vi "Begin.vi"(8 "error in":errorcluster) -> (0 "error out":errorcluster)   [LabVIEW 2018]
doc: "Called before other user functions, this VI is expected to open initial I/O refnums, load in file data, and do all program initialization. Notice that the <B>error out</B> terminal is simply used for data flow. Wiring it to other structures or subVIs ensures that this VI runs first."
uses:
  <vilib>/Rock Robotics/WPI/DriverStation/WPI_DriverStationRobotMode2.ctl
  <vilib>/Rock Robotics/SystemInterfaces/DIO/FPGA_DIOChannel.ctl
  <vilib>/Rock Robotics/SystemInterfaces/DIO/FPGA_DIOPWMChannel.ctl
  <vilib>/Rock Robotics/WPI/Joystick/WPI_JoystickDeviceEnum.ctl
  <vilib>/Rock Robotics/WPI/SafetyOutput/WPI_SafetyOutputConfigMenu.ctl
  <vilib>/Rock Robotics/WPI/Solenoid/WPI_SolenoidChannel.ctl
  <vilib>/Rock Robotics/WPI/Solenoid/WPI_SolenoidValue.ctl
  <vilib>/Rock Robotics/WPI/ThirdParty/Phoenix-LabVIEW/Motor Controller/Controls/CTRE_Phoenix_MotorControl_FeedbackDevice.ctl
  Robot Global Data.vi
  <vilib>/Rock Robotics/Network Tables/NT Write String Array.vi
  <vilib>/Rock Robotics/Network Tables/NT Write Number.vi
  Refnums.vi
  CAN ID's.vi
  <vilib>/Rock Robotics/WPI/RobotDrive/WPI_RobotDriveOpen2MotorWithExistingMotors.vi
  <vilib>/Rock Robotics/WPI/Solenoid/WPI_SolenoidOpenDouble.vi
  <vilib>/Rock Robotics/WPI/Solenoid/WPI_SolenoidSetEnum.vi
  <vilib>/Rock Robotics/WPI/Utilities/WPI_GetSetVariantRefNum.vi
  PID Values.vi
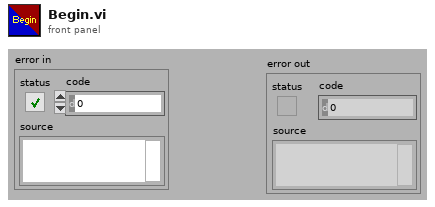
[diagram p1: front panel]
types:
  T1 = typedef "WPI_DriverStationRobotMode2.ctl" = enum16{"Autonomous Disabled", "Autonomous Enabled", "Teleop Disabled", "Teleop Enabled", "Disconnected", "Finish", "Test Disabled", "Test Enabled", "Emergency Stopped"}
  T2 = typedef "WPI_JoystickDeviceEnum.ctl" = enum16{"USB 0", "USB 1", "USB 2", "USB 3", "USB 4", "USB 5"}
  T3 = typedef "FPGA_DIOPWMChannel.ctl" = enum8{"PWM 0", "PWM 1", "PWM 2", "PWM 3", "PWM 4", "PWM 5", "PWM 6", "PWM 7", "PWM 8", "PWM 9", "PWM MXP 0", "PWM MXP 1", "PWM MXP 2", "PWM MXP 3", "PWM MXP 4", "PWM MXP 5", "PWM MXP 6", "PWM MXP 7", "PWM MXP 8", "PWM MXP 9", "Invalid"}
  T4 = typedef "FPGA_DIOChannel.ctl" = enum8{"DIO 0", "DIO 1", "DIO 2", "DIO 3", "DIO 4", "DIO 5", "DIO 6", "DIO 7", "DIO 8", "DIO 9", "DIO MXP 0", "DIO MXP 1", "DIO MXP 2", "DIO MXP 3", "DIO MXP 4", "DIO MXP 5", "DIO MXP 6", "DIO MXP 7", "DIO MXP 8", "DIO MXP 9", "DIO MXP 10", "DIO MXP 11", "DIO MXP 12", "DIO MXP 13", "DIO MXP 14", "DIO MXP 15", "SPI Port CS1", "SPI Port CS2", "SPI Port CS3", "SPI Port MISO", "SPI Port MOSI", "Invalid"}
  T5 = typedef "WPI_SafetyOutputConfigMenu.ctl" = enum16{"Enable", "Disable"}
  T6 = typedef "WPI_SolenoidValue.ctl" = enum16{"Off", "On", "Forward", "Reverse"}
  T7 = typedef "WPI_SolenoidChannel.ctl" = enum8{"Solenoid 0", "Solenoid 1", "Solenoid 2", "Solenoid 3", "Solenoid 4", "Solenoid 5", "Solenoid 6", "Solenoid 7", "Invalid"}
  T8 = typedef "WPI_ServoDeviceRef.ctl" = cluster{"DeviceStatus":errorcluster, "PWM Channel":T3, "DeadBand":T9}
  T9 = typedef "WPI_PWMDeadband.ctl" = cluster{"Name":string, "maxPositivePwm":i32, "minPositivePwm":i32, "centerPwm":i32, "maxNegativePwm":i32, "minNegativePwm":i32, "angularRange":u16}
  T10 = typedef "WPI_JoystickDevRef.ctl" = cluster{"Device":T2}
  T11 = typedef "WPI_DigitalInputDevRef.ctl" = cluster{"DevStatus":errorcluster, "DIO Channel":T4}
  T12 = typedef "WPI_MotorControlDeviceRef.ctl" = cluster{"DeviceStatus":errorcluster, "Type":T13, "PWM":cluster{"PWM Channel":T3, "DeadBand":T9}, "CAN":cluster{"Device Number":u8, "SetOutput VI Ref":variant, "GetOutput VI Ref":variant, "Enable VI Ref":variant, "Disable VI Ref":variant, "Data":variant}, "Invert":bool, "DIO PWM":cluster{"PWM \"Enable\" Channel":T3, "DIOChannel":T4, "PWM Rate":dbl}}
  T13 = typedef "WPI_MotorControlType.ctl" = enum16{"PWM", "CAN", "DIO PWM"}
  T14 = typedef "WPI_RobotDriveDevRef.ctl" = cluster{"DevStatus":errorcluster, "Motors[]":T12[], "Square Inputs":bool, "Max Output":dbl}
  T15 = typedef "WPI_SolenoidDevRef.ctl" = cluster{"DevStatus":errorcluster, "Pneumatics Control Module":u8, "Forward Solenoid Channel":T7, "Reverse Solenoid Channel":T7}
  T16 = typedef "WPI_CompressorDevRef.ctl" = cluster{"DevStatus":errorcluster, "Pneumatics Control Module":u8}
  T17 = cluster{"DriveShifter":T15, "Ouput":T15, "Compressor":T16, "Climb Piston":T15}
  T18 = typedef "CTRE_Phoenix_MotorControl_FeedbackDevice.ctl" = i8
  T19 = cluster{"P":dbl, "I":dbl, "D":dbl, "F":dbl, "I Zone":dbl}
  T20 = cluster{"RightMaster":u8, "RightSlaveA":u8, "RightSlaveB":u8, "LeftMaster":u8, "LeftSlaveA":u8, "LeftSlaveB":u8, "PCM":u8, "PDP":u8, "Intake":u8, "Pivot":u8, "Elevator":u8, "Right Climber":u8, "Left Climber":u8, "Shooter":u8}
  T21 = cluster{"DriveTrain":T14, "LeftDrive":T12, "RightDrive":T12, "Elevator":T12, "Pivot":T12, "Intake":T12, "Right Climber":T12, "Left Climber":T12, "Shooter":T12}
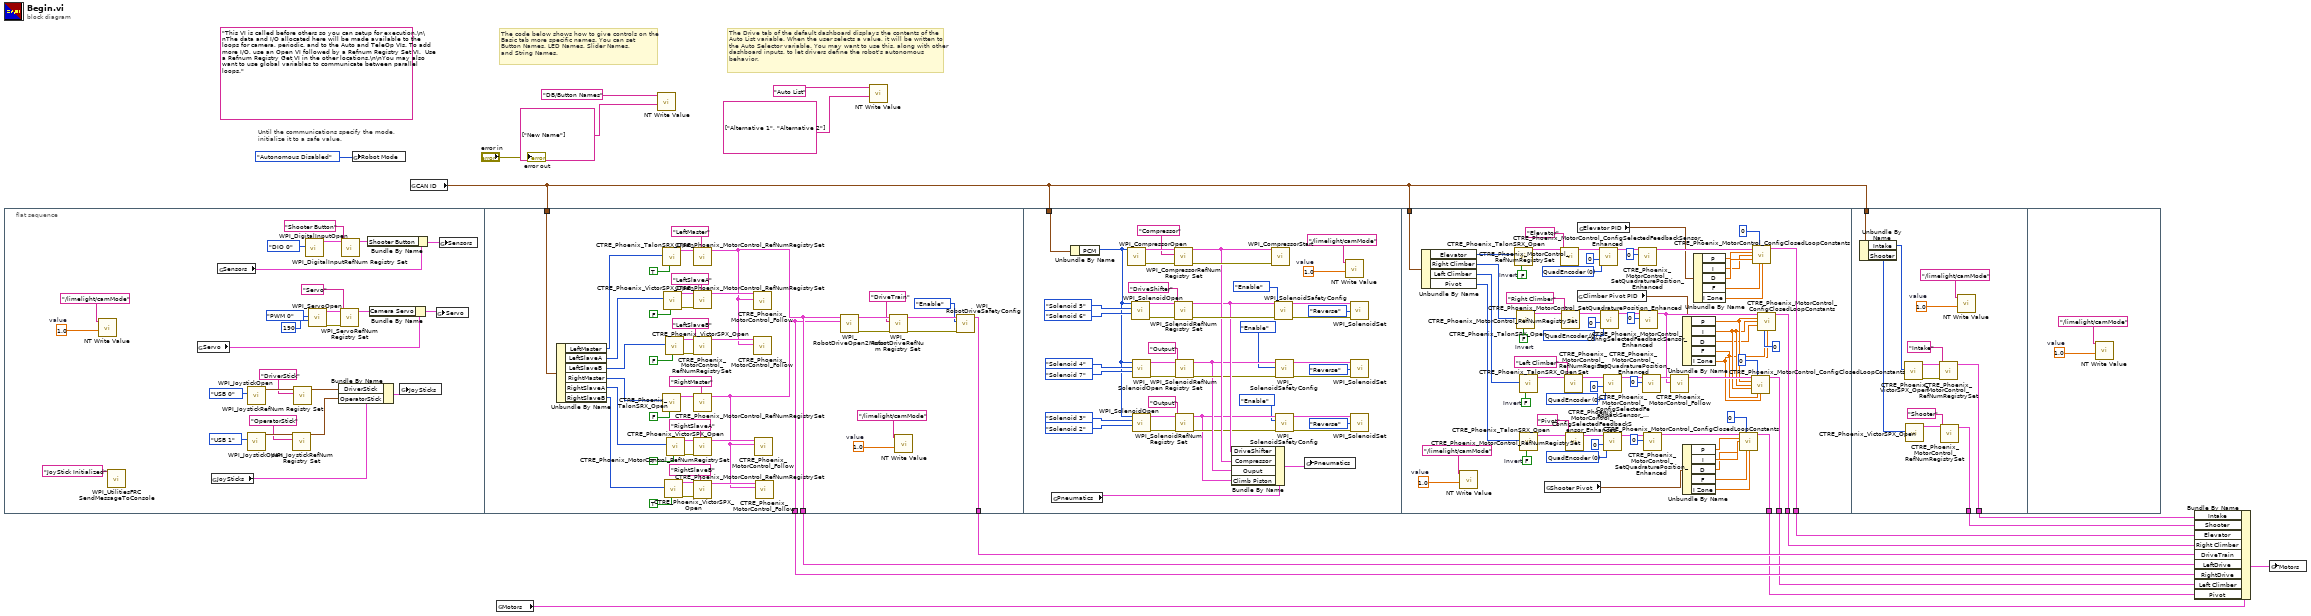
[diagram p0: block diagram]
diagram:
  (unwired) "This VI is called before others so you can setup for execution.\n\nThe data and I/O allocated here will be made available to the loops for camera, periodic, and to the Auto and TeleOp VIs. To add more I/O, use an Open VI followed by a Refnum Registry Set VI.  Use a Refnum Registry Get VI in the other locations.\n\nYou may also want to use global variables to communicate between parallel loops."
  # "The Drive tab of the default dashboard displays the contents of the\nAuto List variable. When the user selects a value, it will be written to\nthe Auto Selector variable. You may want to use this, along with other\ndashboard inputs, to let drivers define the robot's autonomous\nbehavior."
  # "The code below shows how to give controls on the\nBasic tab more specific names. You can set\nButton Names, LED Names, Slider Names,\nand String Names."
  # "Until the communications specify the mode,\ninitialize it to a safe value."
  n1 = flat-sequence {
    tunnel: w3 -> [w69]
    tunnel: [w68] -> w11
    tunnel: [w67] -> w10
    tunnel: [w66] -> w9
    tunnel: w3 -> [w118]
    tunnel: w3 -> [w203]
    tunnel: [w159] -> w7
    tunnel: [w150] -> w6
    tunnel: [w164] -> w5
    tunnel: [w163] -> w4
    tunnel: w3 -> [w210]
    tunnel: [w207] -> w2
    tunnel: [w206] -> w1
    frame #0 {
      w19 = 1.0  # value
      n2 = call-poly <vilib>:"NT Write Value.vi"("Numeric"=w19, "Name"="/limelight/camMode") -> ()  [unwired: 9 in, 1 out]
      n3 = call <vilib>:"WPI_UtilitiesFRC SendMessageToConsole.vi"("Message"="JoyStick Initialized") -> ()  [unwired: 14 in, 1 out]
      n4 = global read "Refnums.vi" "Servo"() -> (w28:cluster{"Camera Servo":T8})
      n5 = global read "Refnums.vi" "JoySticks"() -> (w43:cluster{"DriverStick":T10, "OperatorStick":T10})
      n6 = global read "Refnums.vi" "Sensors"() -> (w31:cluster{"Shooter Button":T11})
      n7 = call <vilib>:"WPI_JoystickOpen.vi"("JoystickDevice"=WPI_JoystickDeviceEnum."USB 1") -> ("JoystickDevRef"=w25:T10)  [unwired: 10 in]
      n8 = call <vilib>:"WPI_JoystickOpen.vi"("JoystickDevice"=WPI_JoystickDeviceEnum."USB 0") -> ("JoystickDevRef"=w45:T10)  [unwired: 10 in]
      n9 = call <vilib>:"WPI_JoystickRefNum Registry Set.vi"("refnum name"="OperatorStick", "JoystickDevRef"=w25) -> ("JoystickDevRef"=w23:T10)  [unwired: 8 in, 1 out]
      n10 = call <vilib>:"WPI_JoystickRefNum Registry Set.vi"("refnum name"="DriverStick", "JoystickDevRef"=w45) -> ("JoystickDevRef"=w42:T10)  [unwired: 8 in, 1 out]
      n11 = call <vilib>:"WPI_DigitalInputOpen.vi"("DIO Channel"=FPGA_DIOChannel."DIO 0") -> ("DigitalInputDevRef"=w38:T11)  [unwired: 9 in, 1 out]
      n12 = call <vilib>:"WPI_ServoOpen.vi"("Angular Range"=u16 190, "PWM Channel"=FPGA_DIOPWMChannel."PWM 0") -> ("error out"=w34:errorcluster, "ServoDeviceRef"=w33:T8)  [unwired: 8 in]
      n13 = Bundle By Name(cluster=w43, "DriverStick"=w42, "OperatorStick"=w23) -> (w41:cluster{"DriverStick":T10, "OperatorStick":T10})
      n14 = call <vilib>:"WPI_ServoRefNum Registry Set.vi"("error in (no error)"=w34, "refnum name"="Servo", "ServoDeviceRef"=w33) -> ("ServoDeviceRef"=w27:T8)  [unwired: 7 in, 1 out]
      n15 = call <vilib>:"WPI_DigitalInputRefNum Registry Set.vi"("refnum name"="Shooter Button", "DigitalInputDevRef"=w38) -> ("DigitalInputDevRef"=w30:T11)  [unwired: 8 in, 1 out]
      n16 = Bundle By Name(cluster=w31, "Shooter Button"=w30) -> (w29:cluster{"Shooter Button":T11})
      n17 = Bundle By Name(cluster=w28, "Camera Servo"=w27) -> (w26:cluster{"Camera Servo":T8})
      n18 = global write "Refnums.vi" "JoySticks"(w41) -> ()
      n19 = global write "Refnums.vi" "Servo"(w26) -> ()
      n20 = global write "Refnums.vi" "Sensors"(w29) -> ()
    }
    frame #1 {
      w46 = 1.0  # value
      n21 = Unbundle By Name(w69) -> ("LeftMaster"=w82:u8, "LeftSlaveA"=w53:u8, "LeftSlaveB"=w52:u8, "RightMaster"=w80:u8, "RightSlaveA"=w51:u8, "RightSlaveB"=w50:u8)
      n22 = call <vilib>:"CTRE_Phoenix_TalonSRX_Open.vi"("Invert"=TRUE, "Device Number"=w82) -> ("CAN Talon SRX Ref"=w83:T12)  [unwired: 8 in, 1 out]
      n23 = call <vilib>:"CTRE_Phoenix_TalonSRX_Open.vi"("Invert"=FALSE, "Device Number"=w80) -> ("CAN Talon SRX Ref"=w81:T12)  [unwired: 8 in, 1 out]
      n24 = call <vilib>:"CTRE_Phoenix_VictorSPX_Open.vi"("Invert"=FALSE, "Device Number"=w53) -> ("error out"=w63:errorcluster, "CAN Talon SRX Ref"=w62:T12)  [unwired: 8 in]
      n25 = call <vilib>:"CTRE_Phoenix_VictorSPX_Open.vi"("Invert"=TRUE, "Device Number"=w50) -> ("error out"=w57:errorcluster, "CAN Talon SRX Ref"=w56:T12)  [unwired: 8 in]
      n26 = call <vilib>:"CTRE_Phoenix_VictorSPX_Open.vi"("Invert"=FALSE, "Device Number"=w52) -> ("error out"=w61:errorcluster, "CAN Talon SRX Ref"=w60:T12)  [unwired: 8 in]
      n27 = call <vilib>:"CTRE_Phoenix_VictorSPX_Open.vi"("Invert"=TRUE, "Device Number"=w51) -> ("error out"=w59:errorcluster, "CAN Talon SRX Ref"=w58:T12)  [unwired: 8 in]
      n28 = call <vilib>:"CTRE_Phoenix_MotorControl_RefNumRegistrySet.vi"("refnum name"="LeftMaster", "PhoenixMotorControlDevRef"=w83) -> ("PhoenixMotorControlDevRef"=w67:T12)  [unwired: 8 in, 1 out]
      n29 = call <vilib>:"CTRE_Phoenix_MotorControl_RefNumRegistrySet.vi"("error in (no error)"=w63, "refnum name"="LeftSlaveA", "PhoenixMotorControlDevRef"=w62) -> ("PhoenixMotorControlDevRef"=w78:T12)  [unwired: 7 in, 1 out]
      n30 = call <vilib>:"CTRE_Phoenix_MotorControl_RefNumRegistrySet.vi"("error in (no error)"=w61, "refnum name"="LeftSlaveB", "PhoenixMotorControlDevRef"=w60) -> ("PhoenixMotorControlDevRef"=w79:T12)  [unwired: 7 in, 1 out]
      n31 = call <vilib>:"CTRE_Phoenix_MotorControl_RefNumRegistrySet.vi"("refnum name"="RightMaster", "PhoenixMotorControlDevRef"=w81) -> ("PhoenixMotorControlDevRef"=w66:T12)  [unwired: 8 in, 1 out]
      n32 = call <vilib>:"CTRE_Phoenix_MotorControl_RefNumRegistrySet.vi"("error in (no error)"=w59, "refnum name"="RightSlaveA", "PhoenixMotorControlDevRef"=w58) -> ("PhoenixMotorControlDevRef"=w77:T12)  [unwired: 7 in, 1 out]
      n33 = call <vilib>:"CTRE_Phoenix_MotorControl_RefNumRegistrySet.vi"("error in (no error)"=w57, "refnum name"="RightSlaveB", "PhoenixMotorControlDevRef"=w56) -> ("PhoenixMotorControlDevRef"=w76:T12)  [unwired: 7 in, 1 out]
      n34 = call <vilib>:"CTRE_Phoenix_MotorControl_Follow.vi"("Master Controller to Follow"=w67, "PhoenixMotorControlDevRef"=w78) -> ()  [unwired: 8 in, 2 out]
      n35 = call <vilib>:"CTRE_Phoenix_MotorControl_Follow.vi"("Master Controller to Follow"=w67, "PhoenixMotorControlDevRef"=w79) -> ()  [unwired: 8 in, 2 out]
      n36 = call <vilib>:"CTRE_Phoenix_MotorControl_Follow.vi"("Master Controller to Follow"=w66, "PhoenixMotorControlDevRef"=w77) -> ()  [unwired: 8 in, 2 out]
      n37 = call <vilib>:"CTRE_Phoenix_MotorControl_Follow.vi"("Master Controller to Follow"=w66, "PhoenixMotorControlDevRef"=w76) -> ()  [unwired: 8 in, 2 out]
      n38 = call-poly <vilib>:"WPI_RobotDriveOpen2Motor.vi"("Right Motor Dev Ref"=w66, "Left Motor Dev Ref"=w67) -> ("error out"=w88:errorcluster, "RobotDriveDevRef"=w87:T14)  [unwired: 3 in, 5 out]
      n39 = call <vilib>:"WPI_RobotDriveRefNum Registry Set.vi"("error in (no error)"=w88, "refnum name"="DriveTrain", "RobotDriveDevRef"=w87) -> ("error out"=w84:errorcluster, "RobotDriveDevRef"=w89:T14)  [unwired: 1 in, 6 out]
      n40 = call-poly <vilib>:"NT Write Value.vi"("Numeric"=w46, "Name"="/limelight/camMode") -> ()  [unwired: 9 in, 1 out]
      n41 = call <vilib>:"WPI_RobotDriveSafetyConfig.vi"("error in (no error)"=w84, "mode"=WPI_SafetyOutputConfigMenu."Enable", "RobotDriveDevRef"=w89) -> ("RobotDriveDevRef"=w68:T14)  [unwired: 7 in, 1 out]
    }
    frame #2 {
      w90 = 1.0  # value
      n42 = global read "Refnums.vi" "Pneumatics"() -> (w122:T17)
      n43 = Unbundle By Name(w118) -> ("PCM"=w92:u8)
      n44 = call <vilib>:"WPI_CompressorOpen.vi"("Pneumatics Control Module (0)"=w92) -> ("CompressorDevRef"=w133:T16, "error out"=w131:errorcluster)  [unwired: 13 in]
      n45 = call-poly <vilib>:"WPI_SolenoidOpen.vi"("Reverse Solenoid Channel"=WPI_SolenoidChannel."Solenoid 6", "Forward Solenoid Channel"=WPI_SolenoidChannel."Solenoid 5", "Pneumatics Control Module (0)"=w92) -> ("error out"=w126:errorcluster, "SolenoidDevRef"=w127:T15)  [unwired: 7 in]
      n46 = call-poly <vilib>:"WPI_SolenoidOpen.vi"("Reverse Solenoid Channel"=WPI_SolenoidChannel."Solenoid 7", "Forward Solenoid Channel"=WPI_SolenoidChannel."Solenoid 4", "Pneumatics Control Module (0)"=w92) -> ("error out"=w112:errorcluster, "SolenoidDevRef"=w113:T15)  [unwired: 7 in]
      n47 = call-poly <vilib>:"WPI_SolenoidOpen.vi"("Reverse Solenoid Channel"=WPI_SolenoidChannel."Solenoid 2", "Forward Solenoid Channel"=WPI_SolenoidChannel."Solenoid 3", "Pneumatics Control Module (0)"=w92) -> ("error out"=w101:errorcluster, "SolenoidDevRef"=w102:T15)  [unwired: 7 in]
      n48 = call <vilib>:"WPI_CompressorRefNum Registry Set.vi"("error in (no error)"=w131, "refnum name"="Compressor", "CompressorDevRef"=w133) -> ("error out"=w130:errorcluster, "CompressorDevRef"=w120:T16)  [unwired: 7 in]
      n49 = call <vilib>:"WPI_SolenoidRefNum Registry Set.vi"("error in (no error)"=w126, "refnum name"="DriveShifter", "SolenoidDevRef"=w127) -> ("error out"=w128:errorcluster, "SolenoidDevRef"=w119:T15)  [unwired: 7 in]
      n50 = call <vilib>:"WPI_SolenoidRefNum Registry Set.vi"("error in (no error)"=w112, "refnum name"="Output", "SolenoidDevRef"=w113) -> ("error out"=w114:errorcluster, "SolenoidDevRef"=w106:T15)  [unwired: 7 in]
      n51 = call <vilib>:"WPI_SolenoidRefNum Registry Set.vi"("error in (no error)"=w101, "refnum name"="Output", "SolenoidDevRef"=w102) -> ("error out"=w103:errorcluster, "SolenoidDevRef"=w94:T15)  [unwired: 7 in]
      n52 = Bundle By Name(cluster=w122, "DriveShifter"=w119, "Compressor"=w120, "Ouput"=w106, "Climb Piston"=w94) -> (w121:T17)
      n53 = call <vilib>:"WPI_CompressorStart.vi"("error in (no error)"=w130, "CompressorDevRef"=w120) -> ()  [unwired: 8 in, 2 out]
      n54 = call <vilib>:"WPI_SolenoidSafetyConfig.vi"("error in (no error)"=w128, "mode"=WPI_SafetyOutputConfigMenu."Enable", "SolenoidDevRef"=w119) -> ("error out"=w117:errorcluster, "SolenoidDevRef"=w116:T15)  [unwired: 7 in]
      n55 = call <vilib>:"WPI_SolenoidSafetyConfig.vi"("error in (no error)"=w114, "mode"=WPI_SafetyOutputConfigMenu."Enable", "SolenoidDevRef"=w106) -> ("error out"=w109:errorcluster, "SolenoidDevRef"=w108:T15)  [unwired: 7 in]
      n56 = call <vilib>:"WPI_SolenoidSafetyConfig.vi"("error in (no error)"=w103, "mode"=WPI_SafetyOutputConfigMenu."Enable", "SolenoidDevRef"=w94) -> ("error out"=w98:errorcluster, "SolenoidDevRef"=w97:T15)  [unwired: 7 in]
      n57 = global write "Refnums.vi" "Pneumatics"(w121) -> ()
      n58 = call-poly <vilib>:"NT Write Value.vi"("Numeric"=w90, "Name"="/limelight/camMode") -> ()  [unwired: 9 in, 1 out]
      n59 = call-poly <vilib>:"WPI_SolenoidSet.vi"("error in (no error)"=w117, "Value"=WPI_SolenoidValue."Reverse", "SolenoidDevRef"=w116) -> ()  [unwired: 7 in, 2 out]
      n60 = call-poly <vilib>:"WPI_SolenoidSet.vi"("error in (no error)"=w109, "Value"=WPI_SolenoidValue."Reverse", "SolenoidDevRef"=w108) -> ()  [unwired: 7 in, 2 out]
      n61 = call-poly <vilib>:"WPI_SolenoidSet.vi"("error in (no error)"=w98, "Value"=WPI_SolenoidValue."Reverse", "SolenoidDevRef"=w97) -> ()  [unwired: 7 in, 2 out]
    }
    frame #3 {
      w134 = 1.0  # value
      w172 = T18 0 items=["QuadEncoder"=0, "Analog"=2, "Tachometer"=4, "Pulse Width Encoded Position"=8, "Sensor Sum (S0 + S1)"=9, "Sensor Difference (D0 - D1)"=10, "Remote Source 0"=11, "Remote Source 1"=12, "Software Emulated"=15] ("Feedback Device")
      w176 = FALSE  # Invert
      w179 = T18 0 items=["QuadEncoder"=0, "Analog"=2, "Tachometer"=4, "Pulse Width Encoded Position"=8, "Sensor Sum (S0 + S1)"=9, "Sensor Difference (D0 - D1)"=10, "Remote Source 0"=11, "Remote Source 1"=12, "Software Emulated"=15] ("Feedback Device")
      w184 = FALSE  # Invert
      w187 = T18 0 items=["QuadEncoder"=0, "Analog"=2, "Tachometer"=4, "Pulse Width Encoded Position"=8, "Sensor Sum (S0 + S1)"=9, "Sensor Difference (D0 - D1)"=10, "Remote Source 0"=11, "Remote Source 1"=12, "Software Emulated"=15] ("Feedback Device")
      w192 = FALSE  # Invert
      w195 = T18 0 items=["QuadEncoder"=0, "Analog"=2, "Tachometer"=4, "Pulse Width Encoded Position"=8, "Sensor Sum (S0 + S1)"=9, "Sensor Difference (D0 - D1)"=10, "Remote Source 0"=11, "Remote Source 1"=12, "Software Emulated"=15] ("Feedback Device")
      w201 = FALSE  # Invert
      n62 = Unbundle By Name(w203) -> ("Elevator"=w199:u8, "Right Climber"=w169:u8, "Left Climber"=w168:u8, "Pivot"=w167:u8)
      n63 = call-poly <vilib>:"NT Write Value.vi"("Numeric"=w134, "Name"="/limelight/camMode") -> ()  [unwired: 9 in, 1 out]
      n64 = call <vilib>:"CTRE_Phoenix_TalonSRX_Open.vi"("Invert"=w201, "Device Number"=w199) -> ("CAN Talon SRX Ref"=w202:T12)  [unwired: 8 in, 1 out]
      n65 = call <vilib>:"CTRE_Phoenix_TalonSRX_Open.vi"("Invert"=w192, "Device Number"=w169) -> ("CAN Talon SRX Ref"=w193:T12)  [unwired: 8 in, 1 out]
      n66 = call <vilib>:"CTRE_Phoenix_TalonSRX_Open.vi"("Invert"=w184, "Device Number"=w168) -> ("CAN Talon SRX Ref"=w185:T12)  [unwired: 8 in, 1 out]
      n67 = call <vilib>:"CTRE_Phoenix_TalonSRX_Open.vi"("Invert"=w176, "Device Number"=w167) -> ("CAN Talon SRX Ref"=w177:T12)  [unwired: 8 in, 1 out]
      n68 = global read "PID Values.vi" "Shooter Pivot"() -> (w151:T19)
      n69 = call <vilib>:"CTRE_Phoenix_MotorControl_RefNumRegistrySet.vi"("refnum name"="Elevator", "PhoenixMotorControlDevRef"=w202) -> ("PhoenixMotorControlDevRef"=w198:T12)  [unwired: 8 in, 1 out]
      n70 = call <vilib>:"CTRE_Phoenix_MotorControl_RefNumRegistrySet.vi"("refnum name"="Right Climber", "PhoenixMotorControlDevRef"=w193) -> ("PhoenixMotorControlDevRef"=w190:T12)  [unwired: 8 in, 1 out]
      n71 = call <vilib>:"CTRE_Phoenix_MotorControl_RefNumRegistrySet.vi"("refnum name"="Left Climber", "PhoenixMotorControlDevRef"=w185) -> ("PhoenixMotorControlDevRef"=w182:T12)  [unwired: 8 in, 1 out]
      n72 = call <vilib>:"CTRE_Phoenix_MotorControl_RefNumRegistrySet.vi"("refnum name"="Pivot", "PhoenixMotorControlDevRef"=w177) -> ("PhoenixMotorControlDevRef"=w175:T12)  [unwired: 8 in, 1 out]
      n73 = global read "PID Values.vi" "Climber Pivot PID"() -> (w142:T19)
      n74 = global read "PID Values.vi" "Elevator PID"() -> (w136:T19)
      n75 = call <vilib>:"CTRE_Phoenix_MotorControl_ConfigSelectedFeedbackSensor_Enhanced.vi"("pidLoopIdx"=0, "Feedback Device"=w195, "PhoenixMotorControlDevRef"=w198) -> ("PhoenixMotorControlDevRef"=w197:T12)  [unwired: 7 in, 1 out]
      n76 = call <vilib>:"CTRE_Phoenix_MotorControl_ConfigSelectedFeedbackSensor_Enhanced.vi"("pidLoopIdx"=0, "Feedback Device"=w187, "PhoenixMotorControlDevRef"=w190) -> ("PhoenixMotorControlDevRef"=w189:T12)  [unwired: 7 in, 1 out]
      n77 = call <vilib>:"CTRE_Phoenix_MotorControl_ConfigSelectedFeedbackSensor_Enhanced.vi"("pidLoopIdx"=0, "Feedback Device"=w179, "PhoenixMotorControlDevRef"=w182) -> ("PhoenixMotorControlDevRef"=w181:T12)  [unwired: 7 in, 1 out]
      n78 = call <vilib>:"CTRE_Phoenix_MotorControl_ConfigSelectedFeedbackSensor_Enhanced.vi"("pidLoopIdx"=0, "Feedback Device"=w172, "PhoenixMotorControlDevRef"=w175) -> ("PhoenixMotorControlDevRef"=w174:T12)  [unwired: 7 in, 1 out]
      n79 = call <vilib>:"CTRE_Phoenix_MotorControl_SetQuadraturePosition_Enhanced.vi"("New Position"=0, "PhoenixMotorControlDevRef"=w197) -> ("PhoenixMotorControlDevRef"=w149:T12)  [unwired: 8 in, 1 out]
      n80 = call <vilib>:"CTRE_Phoenix_MotorControl_SetQuadraturePosition_Enhanced.vi"("New Position"=0, "PhoenixMotorControlDevRef"=w189) -> ("PhoenixMotorControlDevRef"=w165:T12)  [unwired: 8 in, 1 out]
      n81 = call <vilib>:"CTRE_Phoenix_MotorControl_SetQuadraturePosition_Enhanced.vi"("New Position"=0, "PhoenixMotorControlDevRef"=w181) -> ("PhoenixMotorControlDevRef"=w166:T12)  [unwired: 8 in, 1 out]
      n82 = call <vilib>:"CTRE_Phoenix_MotorControl_SetQuadraturePosition_Enhanced.vi"("New Position"=0, "PhoenixMotorControlDevRef"=w174) -> ("PhoenixMotorControlDevRef"=w152:T12)  [unwired: 8 in, 1 out]
      n83 = call <vilib>:"CTRE_Phoenix_MotorControl_Follow.vi"("Master Controller to Follow"=w165, "PhoenixMotorControlDevRef"=w166) -> ("PhoenixMotorControlDevRef"=w162:T12)  [unwired: 8 in, 1 out]
      n84 = Unbundle By Name(w142) -> ("P"=w148:dbl, "I"=w147:dbl, "D"=w146:dbl, "F"=w145:dbl, "I Zone"=w144:dbl)
      n85 = Unbundle By Name(w151) -> ("P"=w157:dbl, "I"=w156:dbl, "D"=w155:dbl, "F"=w154:dbl, "I Zone"=w153:dbl)
      n86 = Unbundle By Name(w136) -> ("P"=w137:dbl, "I"=w138:dbl, "D"=w139:dbl, "F"=w140:dbl, "I Zone"=w141:dbl)
      n87 = call <vilib>:"CTRE_Phoenix_MotorControl_ConfigClosedLoopConstants.vi"("PhoenixMotorControlDevRef"=w152, "slotIdx"=0, "P"=w157, "I"=w156, "D"=w155, "F"=w154, "I Zone"=w153) -> ("PhoenixMotorControlDevRef"=w159:T12)  [unwired: 7 in, 1 out]
      n88 = call <vilib>:"CTRE_Phoenix_MotorControl_ConfigClosedLoopConstants.vi"("PhoenixMotorControlDevRef"=w162, "slotIdx"=0, "P"=w148, "I"=w147, "D"=w147, "F"=w145, "I Zone"=w144) -> ("PhoenixMotorControlDevRef"=w163:T12)  [unwired: 7 in, 1 out]
      n89 = call <vilib>:"CTRE_Phoenix_MotorControl_ConfigClosedLoopConstants.vi"("PhoenixMotorControlDevRef"=w149, "slotIdx"=0, "P"=w137, "I"=w138, "D"=w139, "F"=w140, "I Zone"=w141) -> ("PhoenixMotorControlDevRef"=w150:T12)  [unwired: 7 in, 1 out]
      n90 = call <vilib>:"CTRE_Phoenix_MotorControl_ConfigClosedLoopConstants.vi"("PhoenixMotorControlDevRef"=w165, "slotIdx"=0, "P"=w148, "I"=w147, "D"=w146, "F"=w145, "I Zone"=w144) -> ("PhoenixMotorControlDevRef"=w164:T12)  [unwired: 7 in, 1 out]
    }
    frame #4 {
      w204 = 1.0  # value
      n91 = Unbundle By Name(w210) -> ("Intake"=w208:u8, "Shooter"=w209:u8)
      n92 = call <vilib>:"CTRE_Phoenix_VictorSPX_Open.vi"("Device Number"=w208) -> ("error out"=w215:errorcluster, "CAN Talon SRX Ref"=w214:T12)  [unwired: 9 in]
      n93 = call <vilib>:"CTRE_Phoenix_VictorSPX_Open.vi"("Device Number"=w209) -> ("CAN Talon SRX Ref"=w212:T12)  [unwired: 9 in, 1 out]
      n94 = call <vilib>:"CTRE_Phoenix_MotorControl_RefNumRegistrySet.vi"("error in (no error)"=w215, "refnum name"="Intake", "PhoenixMotorControlDevRef"=w214) -> ("PhoenixMotorControlDevRef"=w206:T12)  [unwired: 7 in, 1 out]
      n95 = call <vilib>:"CTRE_Phoenix_MotorControl_RefNumRegistrySet.vi"("refnum name"="Shooter", "PhoenixMotorControlDevRef"=w212) -> ("PhoenixMotorControlDevRef"=w207:T12)  [unwired: 8 in, 1 out]
      n96 = call-poly <vilib>:"NT Write Value.vi"("Numeric"=w204, "Name"="/limelight/camMode") -> ()  [unwired: 9 in, 1 out]
    }
    frame #5 {
      w216 = 1.0  # value
      n97 = call-poly <vilib>:"NT Write Value.vi"("Numeric"=w216, "Name"="/limelight/camMode") -> ()  [unwired: 9 in, 1 out]
    }
  }
  n98 = global write "Robot Global Data.vi" "Robot Mode"(WPI_DriverStationRobotMode2."Autonomous Disabled" ("Robot Mode")) -> ()
  n99 = global read "CAN ID's.vi" "CAN ID"() -> (w3:T20)
  n100 = global read "Refnums.vi" "Motors"() -> (w12:T21)
  n101 = call-poly <vilib>:"NT Write Value.vi"("String Array"=string[] ["New Name"], "Name"="DB/Button Names") -> ()  [unwired: 9 in, 1 out]
  n102 = call-poly <vilib>:"NT Write Value.vi"("String Array"=string[] ["Alternative 1", "Alternative 2"], "Name"="Auto List") -> ()  [unwired: 9 in, 1 out]
  n103 = Bundle By Name(cluster=w12, "Intake"=w1, "Shooter"=w2, "Elevator"=w6, "Right Climber"=w5, "DriveTrain"=w11, "LeftDrive"=w10, "RightDrive"=w9, "Left Climber"=w4, "Pivot"=w7) -> (w8:T21)
  n104 = global write "Refnums.vi" "Motors"(w8) -> ()
  "error out" <- "error in"
